vi "Messaging EnQ Multiline String.vi"(5 "Command(s)":string, 6 "@Front?":bool, 8 "error in (no error)":errorcluster) -> (0 "error out":errorcluster)   [LabVIEW 2019, in "GUI.lvlib"]
doc: "Enqueues <b>Command(s)</b> to the Queues. The commands are EOL delimted and the string after the \">>\" will be comma delimited as data available to the case.\n\nOptionally enqueue at the <b>Front?</b>"
uses:
  GUI.lvlib
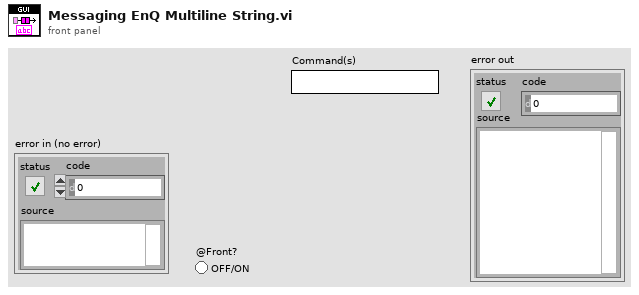
[diagram p1: front panel]
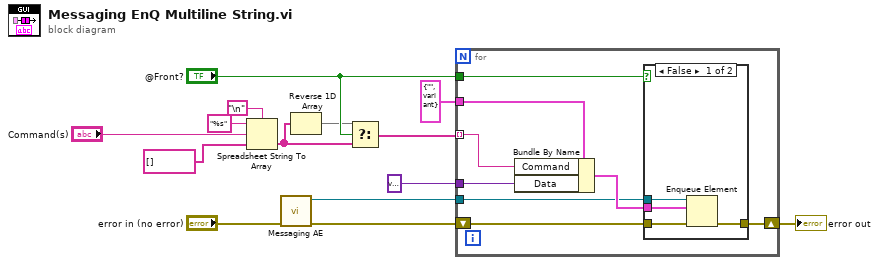
[diagram p0: block diagram]
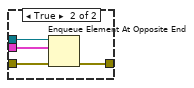
[diagram p2: hidden frame]
diagram:
  n1 = Spreadsheet String To Array(delimiter (Tab)="\n", format string="%s", spreadsheet string="Command(s)", array type (2D Dbl)=string[] []) -> (array=w1:string[])
  n2 = call "Messaging AE.vi"("Error In"="error in (no error)") -> ("Error Out"=w7:errorcluster, "queue out"=w6:refnum<queue>)  [unwired: 9 in]
  n3 = Reverse 1D Array(array=w1) -> (reversed array=w2:string[])
  n4 = Select(t=w2, s="@Front?", f=w1) -> (s? t:f=w4:string[])
  n5 = for {
    tunnel: variant ("Data") -> [w22]
    tunnel: w4 -> [w21] mode=indexing
    shift-right: [w18] -> w12
    shift-left: w7 -> [w17]
    tunnel: "@Front?" -> [w16]
    tunnel: w6 -> [w19]
    tunnel: cluster{"Command":string, "Data":variant} {"Command"="", "Data"=variant} ("Message Data") -> [w15]
    n6 = Bundle By Name(cluster=w15, "Command"=w21, "Data"=w22) -> (w20:cluster{"Command":string, "Data":variant})
    n7 = case shown="False" w16 {
      tunnel: w20 -> [w26 w30]
      tunnel: w19 -> [w25 w29]
      tunnel: [w24 w27] -> w18
      tunnel: w17 -> [w23 w28]
      frame False {
        n8 = Enqueue Element(queue=w25, element=w26, error in (no error)=w23) -> (error out=w24:errorcluster)  [unwired: 1 in, 2 out]
      }
      frame True {
        n9 = Enqueue Element At Opposite End(queue=w29, element=w30, error in (no error)=w28) -> (error out=w27:errorcluster)  [unwired: 1 in, 2 out]
      }
    }
  }
  "error out" <- w12
